vi "GetConfigOld.vi"(8 "error in (no error)":errorcluster, 11 "QuickSilver in":refnum<class "QuickSilver.lvclass">) -> (0 "error out":errorcluster, 3 "QuickSilver out":refnum<class "QuickSilver.lvclass">)   [LabVIEW 2011]
uses:
  Global Coude.vi
  QuickSilver.lvclass
panel:
  out "String":string
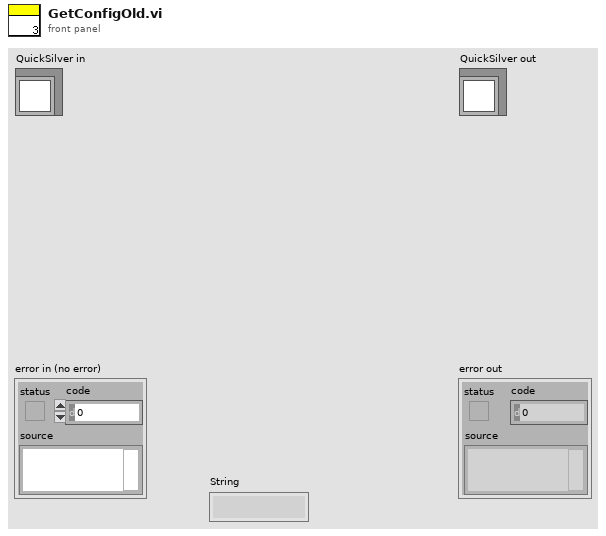
[diagram p1: front panel]
types:
  T1 = cluster{"Mec ID":void, "VISA Mec":void, "Mec PosLimit":void, "Mec NegLimit":void, "Mec Factor":void, "Mec Speed":void, "Mec Acceleration":void, "MecOffset":void, "MecTargets":void, "MecEnabled":void, "Mec Target":void}
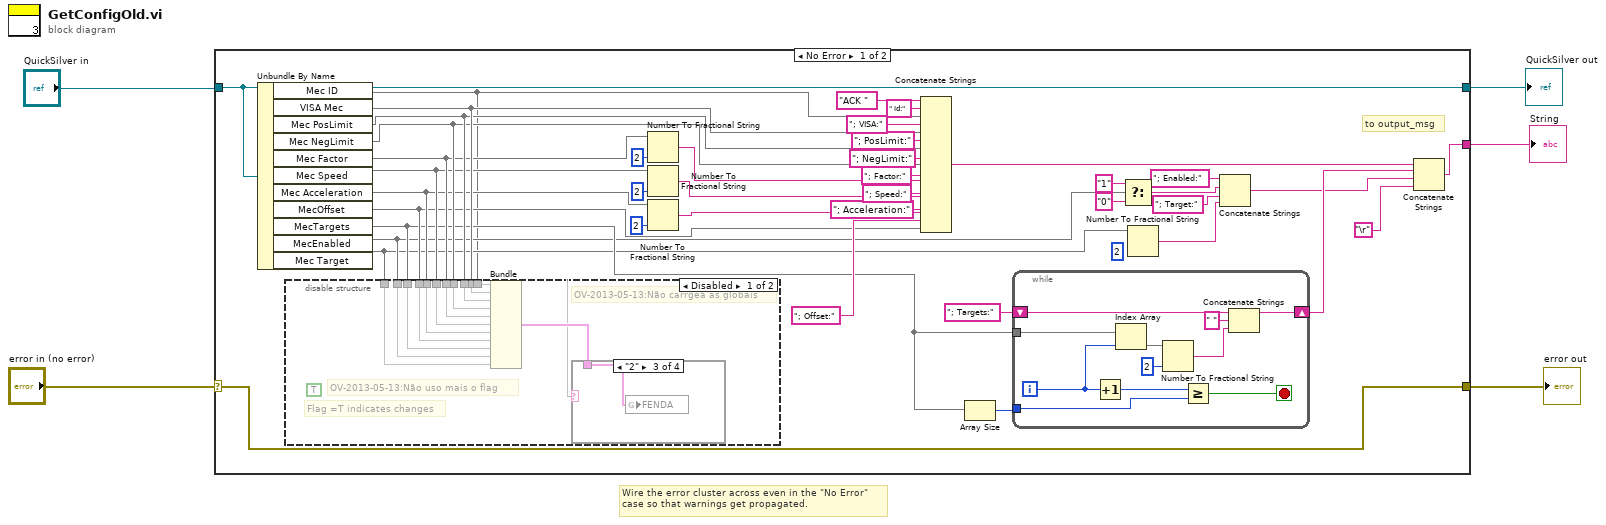
[diagram p0: block diagram]
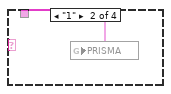
[diagram p3: hidden frame]
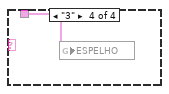
[diagram p4: hidden frame]
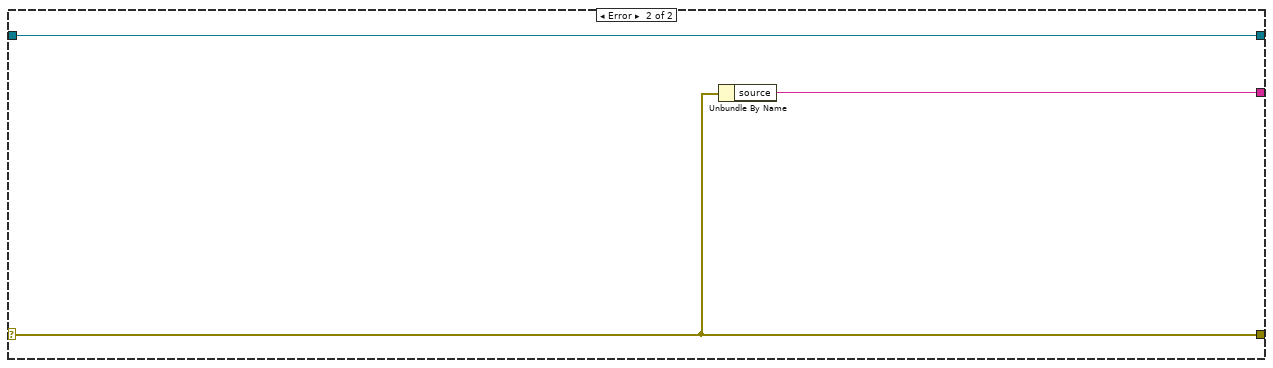
[diagram p6: hidden frame]
diagram:
  # "Wire the error cluster across even in the \"No Error\"\ncase so that warnings get propagated."
  n1 = case shown="No Error" "error in (no error)" {
    selector: "error in (no error)" -> [w25 w74]
    tunnel: [w25 w74] -> w2
    tunnel: [w46 w75] -> w1
    tunnel: "QuickSilver in" -> [w46 w75]
    tunnel: [w26 w73] -> w5
    frame No Error {
      (unwired) i16 2 ("precision (6)")
      # "to output_msg"
      n2 = Unbundle By Name(w46) -> ("Mec ID"=w6, "VISA Mec"=w16, "Mec PosLimit"=w15, "Mec NegLimit"=w14, "Mec Factor"=w13, "Mec Speed"=w12, "Mec Acceleration"=w11, "MecOffset"=w10, "MecTargets"=w9, "MecEnabled"=w8, "Mec Target"=w7)
      n3 = disable-structure shown="Disabled" {
        disable-tunnel: w16 -> [w58 _]
        disable-tunnel: w15 -> [w57 _]
        disable-tunnel: w14 -> [w56 _]
        disable-tunnel: w13 -> [w55 _]
        disable-tunnel: w12 -> [w54 _]
        disable-tunnel: w11 -> [w53 _]
        disable-tunnel: w10 -> [w52 _]
        disable-tunnel: w9 -> [w51 _]
        disable-tunnel: w8 -> [w50 _]
        disable-tunnel: w7 -> [w49 _]
        disable-tunnel: w6 -> [w47 _]
        frame Disabled {
          (unwired) TRUE
          # "OV-2013-05-13:Não carrgea as globais"
          # "OV-2013-05-13:Não uso mais o flag"
          # "Flag =T indicates changes"
          n4 = Bundle("Mec ID"=w47, "VISA Mec"=w58, "Mec PosLimit"=w57, "Mec NegLimit"=w56, "Mec Factor"=w55, "Mec Speed"=w54, "Mec Acceleration"=w53, "MecOffset"=w52, "MecTargets"=w51, "MecEnabled"=w50, "Mec Target"=w49) -> (w48:T1)  [unwired: 1 out]
          n5 = case shown="\"2\"" w47 {
            tunnel: w48 -> [_ w59 w60 w61]
            frame Default {
            }
            frame "1" {
              n6 = global write "Global Coude.vi" "PRISMA"(w59) -> ()
            }
            frame "2" {
              n7 = global write "Global Coude.vi" "FENDA"(w60) -> ()
            }
            frame "3" {
              n8 = global write "Global Coude.vi" "ESPELHO"(w61) -> ()
            }
          }
        }
        frame Enabled {
        }
      }
      n9 = Number To Fractional String(number=w13, precision (6)=i16 2) -> (F-format string=w43:string)  [unwired: 2 out]
      n10 = Number To Fractional String(number=w12, precision (6)=i16 2) -> (F-format string=w44:string)  [unwired: 2 out]
      n11 = Number To Fractional String(number=w11, precision (6)=i16 2) -> (F-format string=w45:string)  [unwired: 2 out]
      n12 = Concatenate Strings("ACK " ("string"), " Id:" ("string"), w6, "; VISA:" ("string"), w16, "; PosLimit:" ("string"), w15, "; NegLimit:" ("string"), w14, "; Factor:" ("string"), w43, "; Speed:" ("string"), w44, "; Acceleration:" ("string"), w45, "; Offset:" ("string"), w10) -> (w30:string)
      n13 = Array Size(array=w9) -> (size(s)=w32:i32)
      n14 = while {
        tunnel: w9 -> [w72]
        shift-right: [w71] -> w31
        shift-left: "; Targets:" ("string") -> [w70]
        tunnel: w32 -> [w68]
        i -> [w66]
        stop <- w67 stop-if-true
        n15 = Increment(x=w66) -> (x+1=w65:i32)
        n16 = Index Array(array=w72, index=w66) -> (element=w62)
        n17 = Number To Fractional String(number=w62, precision (6)=i16 2) -> (F-format string=w64:string)  [unwired: 2 out]
        n18 = Greater Or Equal?(x=w65, y=w68) -> (x >= y?=w67:bool)
        n19 = Concatenate Strings(w70, " " ("string"), w64) -> (w71:string)
      }
      n20 = Select(t="1", s=w8, f="0") -> (s? t:f=w21:string)
      n21 = Number To Fractional String(number=w7) -> (F-format string=w19:string)  [unwired: 3 out]
      n22 = Concatenate Strings("; Enabled:" ("string"), w21, "; Target:" ("string"), w19) -> (w18:string)
      n23 = Concatenate Strings(w30, w31, w18, "\r") -> (w26:string)
    }
    frame Error {
      n24 = Unbundle By Name(w74) -> ("source"=w73:string)
    }
  }
  "error out" <- w2
  "QuickSilver out" <- w1
  "String" <- w5
